vi "Flush Queue.vi"(8 "error in":errorcluster, 11 "QDMH in":refnum<class "QDMH.lvclass">) -> (0 "error out":errorcluster, 2 "Flushed elements":T1[](array[typedef]), 3 "QDMH out":refnum<class "QDMH.lvclass">)   [LabVIEW 2023, in "QDMH.lvlib" / "QDMH.lvclass"]
uses:
  QDMH.lvclass
  Custom Controls/QDMH Message.ctl
  QDMH.lvclass/QDMH.ctl
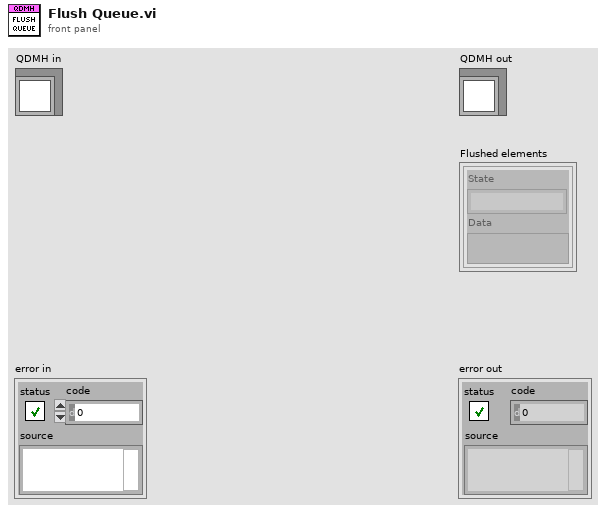
[diagram p1: front panel]
types:
  T1 = typedef "QDMH.lvlib/QDMH.lvclass/QDMH Message.ctl" = cluster{"State":string, "Data":variant}
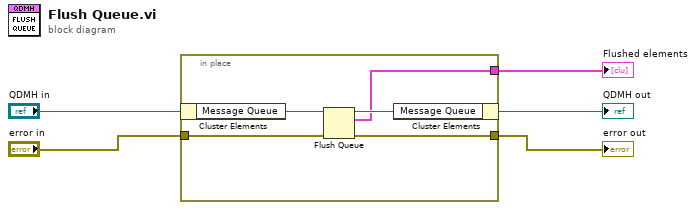
[diagram p0: block diagram]
diagram:
  n1 = in-place {
    in-place-border: [w8] -> w1
    in-place-border: "error in" -> [w7]
    in-place-border: [w6] -> w3
    n2 = in-place-cluster #1("QDMH in") -> ("Message Queue"=w10:refnum<queue>)
    n3 = Flush Queue(queue=w10, error in (no error)=w7) -> (queue out=w9:refnum<queue>, remaining elements=w8:T1[], error out=w6:errorcluster)
    n4 = in-place-cluster #1("Message Queue"=w9) -> (→"QDMH out":refnum<class "QDMH.lvclass">)
  }
  "error out" <- w3
  "Flushed elements" <- w1
